vi "ExCircNframeBigBufQ.vi"() -> ()   [LabVIEW 2010]
uses:
  Open-Close/CamHandle.vi
panel:
  out "ready to \nstart":bool
  in  "Start collection":bool
  in  "Timing Mode":u32(ring)=1 items=["N/A", "Timed Mode/Free run", "Trigger First (only PM)", "Strobed/Ext Sync", "Bulb Mode (PM only)", "Variable Timed mode (PM only)", "Flash Mode (only some PM)"]
  in  "Number of Images":u32=1 min=1 step=1
  in  "Exposure":dbl min=0.0 step=0.001 format="%.3f"
  out "error out":errorcluster
  in  "error in (no error)":errorcluster
  # "ExCircNframeBigBuf:\nThis example collects, displays, and saves in \na .spe file the number of images selected. This \nexample requires the camera have circular \nbuffers capability. \nFirst this example creates an array of image \nhandles. It then collects data into this array.\nFinally it displays and saves all the images."
  # "NOTICE\n\nTHIS VI USES A GLOBAL CAMERA HANDLE\n\nTHE VI EXOPENGLOBALCAM.VI MUST BE\nRUN AT THE START OF THE WORK SESSION.\nTHE CAMERA WILL REMAIN OPENED.\n\nTHE VI EXCLOSEGLOBALCAM.VI MUST\nBE RUN BEFORE LEAVING LABVIEW."
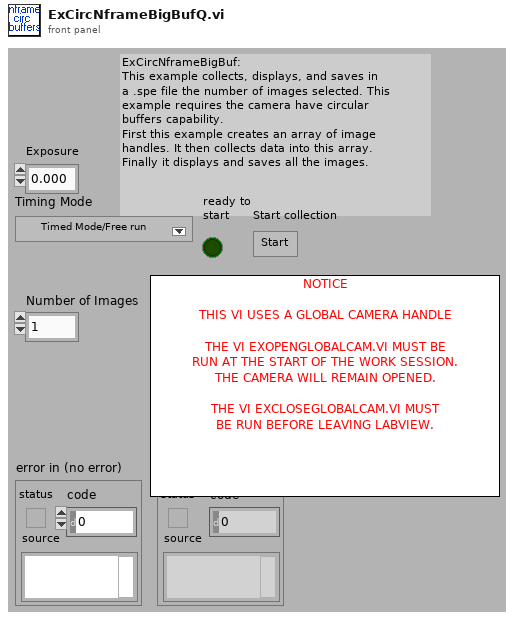
[diagram p1: front panel]
types:
  T1 = cluster{"acquire focus mode":u32, "Exposure":dbl, "Number of Images":u32, "Software accumulation":u32}
  T2 = cluster{"Camera Handle":u32, "Pulser Handle":u32, "File Handle":u32, "Display Handle":u32, "Image Handle":u32}
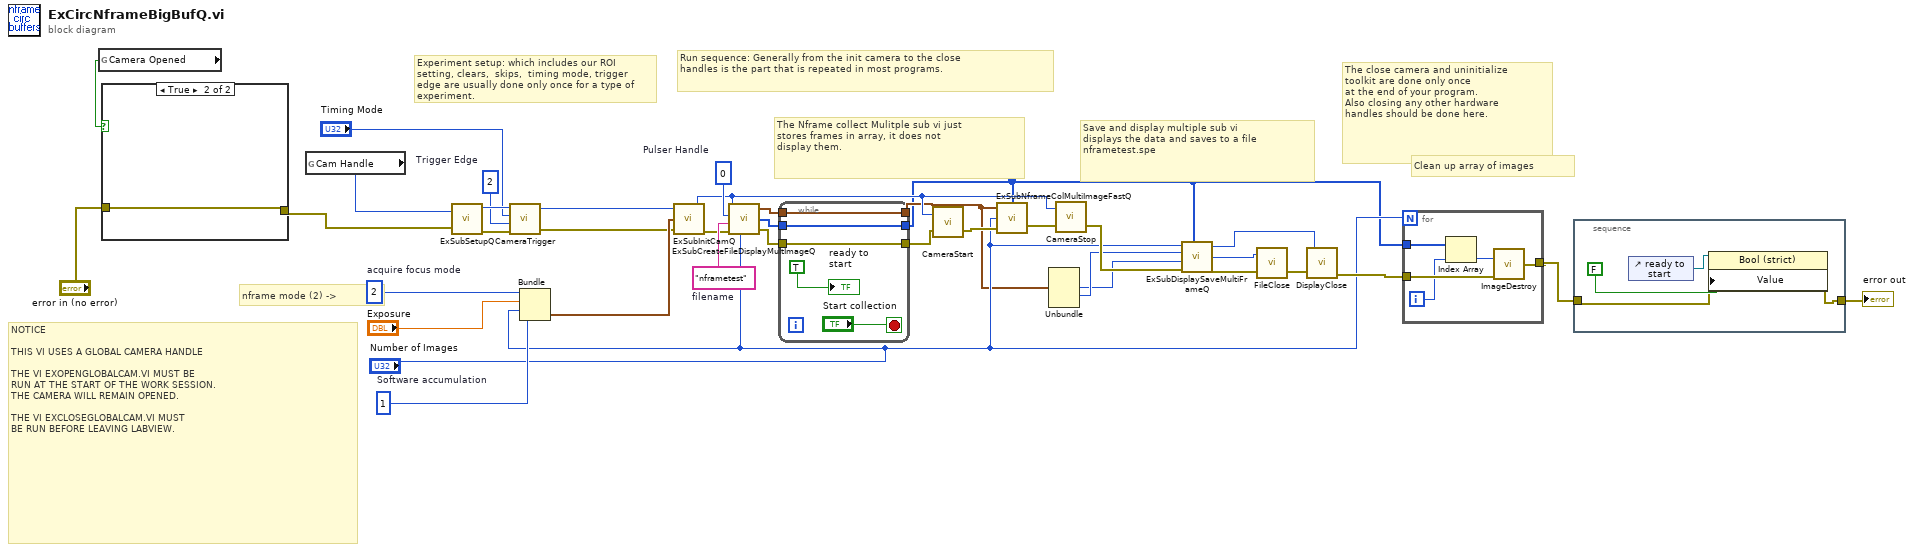
[diagram p0: block diagram]
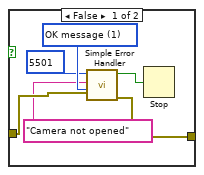
[diagram p2: hidden frame]
diagram:
  w28 = u32 0  # Pulser Handle
  w29 = u32 2  # Trigger Edge
  w31 = u32 2  # acquire focus mode
  w30 = u32 1  # Software accumulation
  w37 = "nframetest"  # filename
  # "NOTICE\n\nTHIS VI USES A GLOBAL CAMERA HANDLE\n\nTHE VI EXOPENGLOBALCAM.VI MUST BE\nRUN AT THE START OF THE WORK SESSION.\nTHE CAMERA WILL REMAIN OPENED.\n\nTHE VI EXCLOSEGLOBALCAM.VI MUST\nBE RUN BEFORE LEAVING LABVIEW."
  # "Clean up array of images"
  # "Save and display multiple sub vi\ndisplays the data and saves to a file\nnframetest.spe"
  # "The Nframe collect Mulitple sub vi just \nstores frames in array, it does not \ndisplay them."
  # "The close camera and uninitialize\ntoolkit are done only once\nat the end of your program.\nAlso closing any other hardware \nhandles should be done here."
  # "Run sequence: Generally from the init camera to the close \nhandles is the part that is repeated in most programs."
  # "Experiment setup: which includes our ROI setting, clears,  skips,  timing mode, trigger edge are usually done only once for a type of experiment."
  # "nframe mode (2) ->"
  n1 = global read "CamHandle.vi" "Camera Opened"() -> (w4:bool)
  n2 = case shown="True" w4 {
    tunnel: "error in (no error)" -> [w42 w44]
    tunnel: [w41 w44] -> w2
    frame False {
      w43 = u16 1 items=["no dialog", "OK message", "continue or stop message"] ("type of dialog (OK msg:1)")
      n3 = call <vilib>:"Simple Error Handler.vi"("error code (no error:0)"=5501, "error source (\" \")"="Camera not opened", "type of dialog (OK msg:1)"=w43, "error in (no error)"=w42) -> ("error?"=w39:bool, "error out"=w41:errorcluster)  [unwired: 1 in, 3 out]
      n4 = Stop(stop? (T)=w39) -> ()
    }
    frame True {
    }
  }
  n5 = global read "CamHandle.vi" "Cam Handle"() -> (w1:u32)
  n6 = call "ExSubSetupQ.vi"("error in (no error)"=w2, "Camera Handle"=w1) -> ("error out"=w32:errorcluster, "Camera Handle"=w33:u32)
  n7 = call <userlib>:"CameraTrigger.vi"("error in"=w32, "Trigger Edge"=w29, "Timing Mode"="Timing Mode", "Camera Handle"=w33) -> ("error out"=w6:errorcluster, "Camera Handle"=w7:u32)
  n8 = Bundle("acquire focus mode"=w31, "Exposure"="Exposure", "Number of Images"="Number of Images", "Software accumulation"=w30) -> (w35:T1)  [unwired: 1 in]
  n9 = call "ExSubInitCamQ.vi"("error in (no error)"=w6, "Camera Information"=w35, "Camera Handle"=w7) -> ("error out"=w34:errorcluster, "Camera Handle"=w25:u32)
  n10 = call "ExSubCreateFileDisplayMultImageQ.vi"("Camera Handle"=w25, "Pulser Handle"=w28, "File and Display Name"=w37, "error in (no error)"=w34, "Number of Images"="Number of Images") -> ("Handles Out"=w14:T2, "Array"=w10:u32[], "error out"=w12:errorcluster)
  n11 = while {
    tunnel: w14 -> [w49]
    tunnel: [w49] -> w13
    tunnel: w12 -> [w48]
    tunnel: [w48] -> w11
    tunnel: w10 -> [w47]
    tunnel: [w47] -> w9
    stop <- "Start collection" stop-if-true
    "ready to \nstart" <- TRUE
  }
  n12 = call <userlib>:"CameraStart.vi"("error in"=w11, "Camera Handle"=w25) -> ("error out"=w27:errorcluster)  [unwired: 1 out]
  n13 = call "ExSubNframeColMultiImageFastQ.vi"("image handles"=w9, "error in (no error)"=w27, "Number of Images"="Number of Images", "Handle Cluster"=w13) -> ("error out"=w26:errorcluster)  [unwired: 1 out]
  n14 = Unbundle(w13) -> ("File Handle"=w21:u32, "Display Handle"=w22:u32)  [unwired: 3 out]
  n15 = call <userlib>:"CameraStop.vi"("error in"=w26, "Camera Handle"=w25) -> ("error out"=w23:errorcluster)  [unwired: 1 out]
  n16 = call "ExSubDisplaySaveMultiFrameQ.vi"("Number of Images"="Number of Images", "Display Handle"=w22, "file handle"=w21, "error in (no error)"=w23, "Data handles"=w9) -> ("Display Handle"=w16:u32, "file Handle"=w17:u32, "error out"=w18:errorcluster)
  n17 = call <userlib>:"FileClose.vi"("error in"=w18, "File Handle"=w17) -> ("error out"=w20:errorcluster)
  n18 = call <userlib>:"DisplayClose.vi"("error in"=w20, "Display Handle"=w16) -> ("error out"=w19:errorcluster)
  n19 = for {
    N: "Number of Images" -> [_]
    tunnel: w19 -> [w54]
    tunnel: [w53] -> w8
    tunnel: w9 -> [w51]
    i -> [w52]
    n20 = Index Array(array=w51, index=w52) -> (element=w50:u32)
    n21 = call <userlib>:"ImageDestroy.vi"("error in"=w54, "Data handle"=w50) -> ("error out"=w53:errorcluster)
  }
  n22 = stacked-sequence {
    tunnel: w8 -> [w56]
    tunnel: [w55] -> w3
    frame #0 {
      n23 = control-ref of="ready to \nstart"() -> (w58:refnum<vi>)
      n24 = property class="Bool (strict)"(reference=w58, error in=w56, "Value"=FALSE) -> (error out=w55:errorcluster)  [unwired: 1 out]
    }
  }
  "error out" <- w3
